vi "ActFollowAbsoluteTrajectory.vi"(10 "Trajectory":T1 {"States"."POSE"."ROTATION"."SIN" format="%13.4f"; "States"."POSE"."ROTATION"."COS" format="%13.4f"; "States"."POSE"."ROTATION"."VALUE" format="%13.4f"; "States"."POSE"."TRANSLATION"."Y" format="%14.3f"; "States"."POSE"."TRANSLATION"."X" format="%14.3f"; "TotalTImeSecs" format="%20.3f"}, 11 "FirstTime":bool) -> (0 "Done":bool, 1 "ASpeedDemand":dbl, 2 "YSpeedDemand":dbl, 3 "XSpeedDemand":dbl)   [LabVIEW 2023]
uses:
  <vilib>/Rock Robotics/WPI/ThirdParty/JAS_Junk/TrajLib/TypeDef/TRAJECTORY.ctl
  <vilib>/Rock Robotics/WPI/ThirdParty/JAS_Junk/TrajLib/TypeDef/TRAJ_STATE.ctl
  <vilib>/Rock Robotics/WPI/ThirdParty/JAS_Junk/TrajLib/TypeDef/POSE2D.ctl
  <vilib>/Rock Robotics/WPI/ThirdParty/JAS_Junk/TrajLib/TypeDef/TRANSLATION2D.ctl
  <vilib>/Rock Robotics/WPI/ThirdParty/JAS_Junk/TrajLib/TypeDef/ROTATION2D.ctl
  Autonomous/TrajectoryOrientation.ctl
  Vision/VisionGlobal.vi
  <vilib>/Rock Robotics/WPI/ThirdParty/JAS_Junk/TrajLib/Trajectory_Library.lvlib
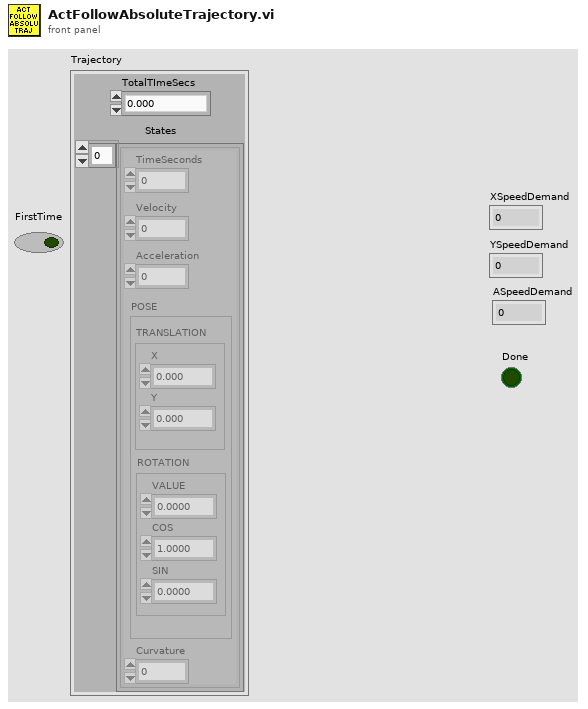
[diagram p1: front panel]
types:
  T1 = typedef "Trajectory_Library.lvlib/TRAJECTORY.ctl" = cluster{"TotalTImeSecs":dbl, "States":T2[]}
  T2 = typedef "Trajectory_Library.lvlib/TRAJ_STATE.ctl" = cluster{"TimeSeconds":dbl, "Velocity":dbl, "Acceleration":dbl, "POSE":T3, "Curvature":dbl}
  T3 = typedef "Trajectory_Library.lvlib/POSE2D.ctl" = cluster{"TRANSLATION":T4, "ROTATION":T5}
  T4 = typedef "Trajectory_Library.lvlib/TRANSLATION2D.ctl" = cluster{"X":dbl, "Y":dbl}
  T5 = typedef "Trajectory_Library.lvlib/ROTATION2D.ctl" = cluster{"VALUE":dbl, "COS":dbl, "SIN":dbl}
  T6 = typedef "TrajectoryOrientation.ctl" = enum16{"SameOrientation", "RotateToEndOrientation"}
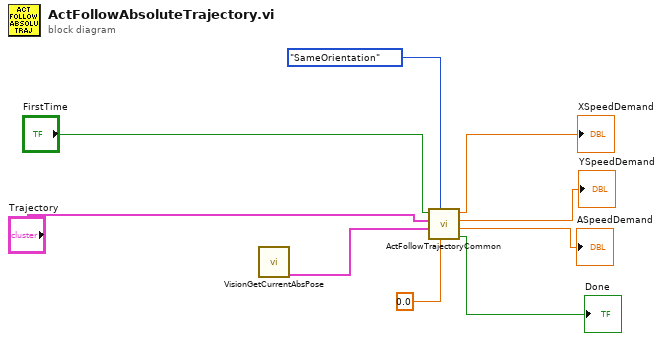
[diagram p0: block diagram]
diagram:
  n1 = call "VisionGetCurrentAbsPose.vi"() -> ("Current ABS Pose"=w3:T3)  [unwired: 9 in]
  n2 = call "ActFollowTrajectoryCommon.vi"("End Orientation"=0.0, "Orientation"=TrajectoryOrientation."SameOrientation", "currentPose"=w3, "Trajectory"="Trajectory", "FirstTime"="FirstTime") -> ("Done"=→"Done":bool, "vAngularDemand"=→"ASpeedDemand":dbl, "vYSpeedDemand"=→"YSpeedDemand":dbl, "vXSpeedDemand"=→"XSpeedDemand":dbl)  [unwired: 3 in]
